vi "Calibration - Conductivity.vi"() -> ()   [LabVIEW 2016]
uses:
  calibration states.ctl
panel:
  in  "Highpoint":i32=1413 min=0
  in  "Lowpoint":i32=84 min=0
  in  "Calibrate3":bool
  out "Read indicator":bool
  out "Reading, uS/cm":dbl
  in  "Calibrate2":bool
  out "Status":string
  in  "Cancel":bool
  in  "Calibrate1":bool
  # "ATLAS SCIENTIFIC\nCONDUCTIVITY SENSOR CALIBRATION"
  # "Temperature has a significant effect on conductivity readings. The EZO Conductivity circuit has its temperature compensation set to 25C as the default. If the calibration solution is not within 5C of 25 C, check the temperature chart on the side of the calibration bottle, and calibrate to that value.\n\nLow point/single point calibration:\n1. Pour a small amount of the calibration solution into a cup. Shake the probe to make sure you do not have trapped air bubbles in the sensing area. \n2. You should see readings that are off by 1 – 40% from the stated value of the calibration solution. Wait for readings to stabilize (small movement from one reading to the next is normal).\n3. Once the readings stabilize, issue the \"Calibrate lowpoint\" command. Readings will NOT change - the calibration is not yet complete.\n\nHigh point calibration:\n1. Shake the probe to remove trapped air and adjust the temperature as done in the previous step.\n2. Once the readings have stabilized issue the \"Calibrate highpoint\" command. - Readings will change, calibration complete."
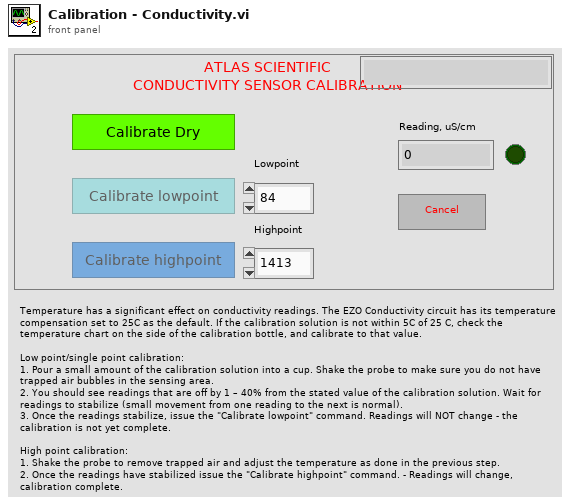
[diagram p1: front panel]
types:
  T1 = enum32{"Invalid", "Standard", "Closed", "Hidden", "Minimized", "Maximized"}
  T2 = typedef "Visa com cluster def (subVI).ctl" = cluster{"Sensor":string, "VISA resource name":refnum<visa-resource-name>, "error in/out":errorcluster, "bytes read":u32, "Com found ?":bool}
  T3 = typedef "calibration states.ctl" = string
  T4 = enum8{"Enabled", "Disabled", "Disabled and Grayed Out"}
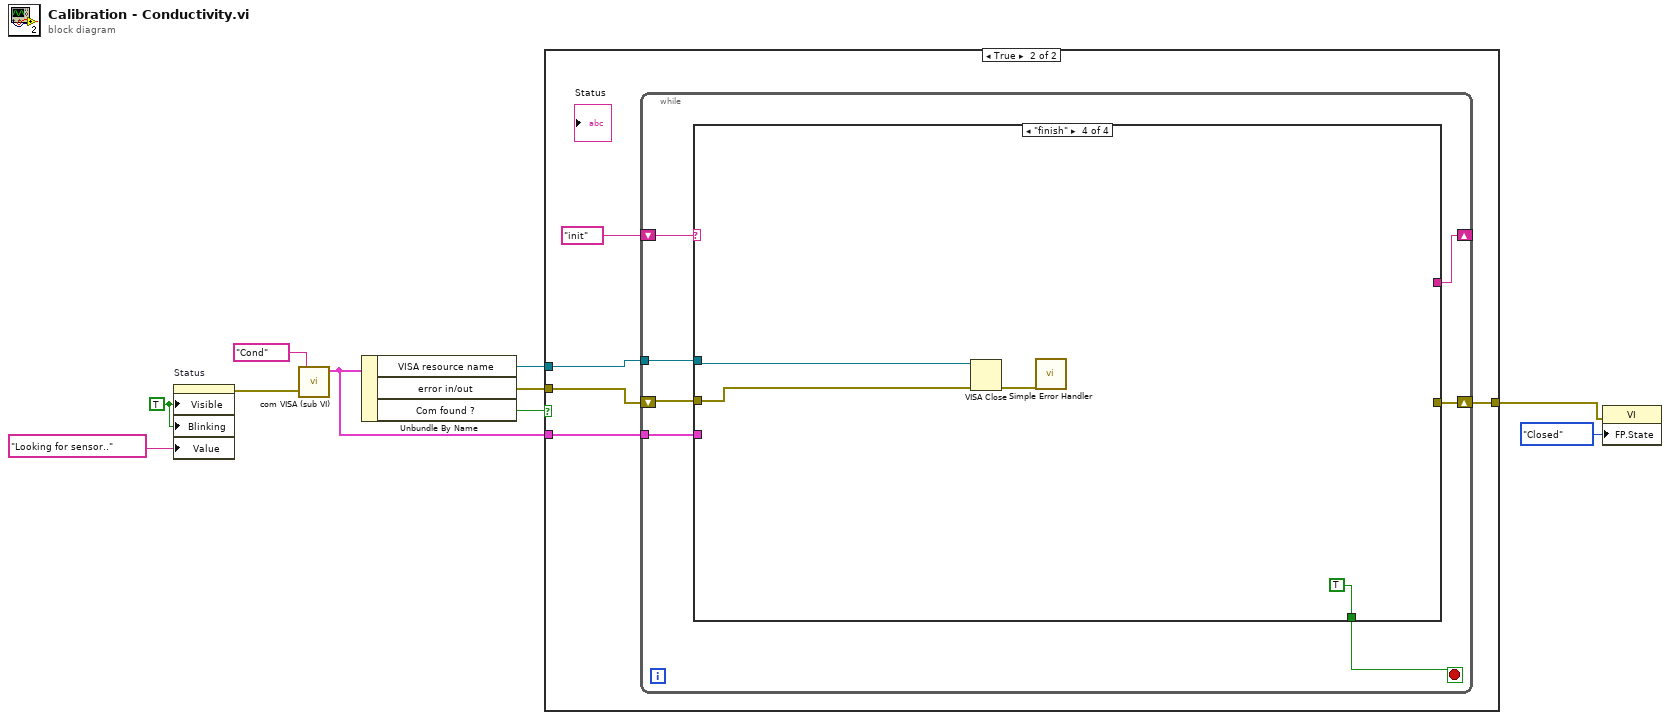
[diagram p0: block diagram]
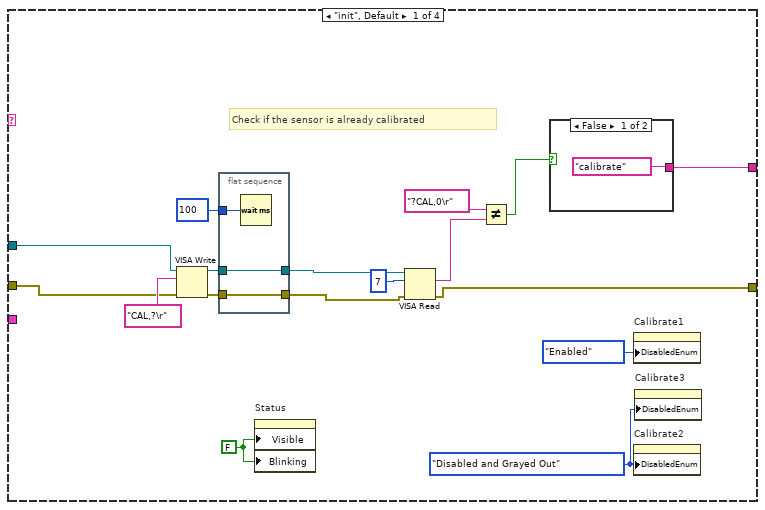
[diagram p3: hidden frame]
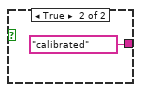
[diagram p4: hidden frame]
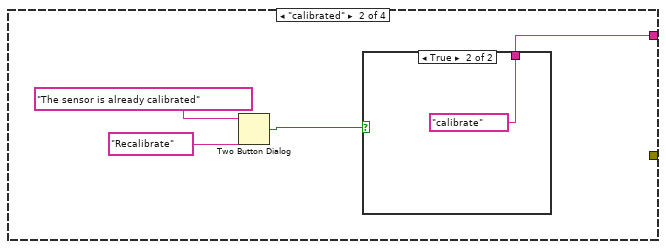
[diagram p5: hidden frame]
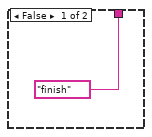
[diagram p6: hidden frame]
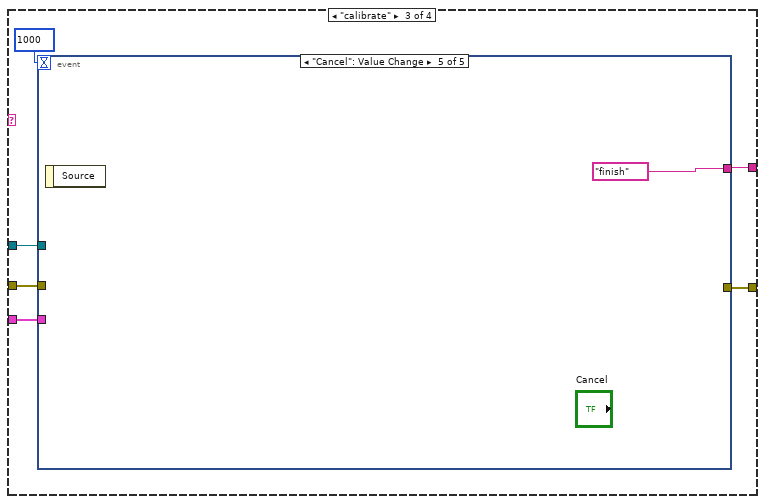
[diagram p7: hidden frame]
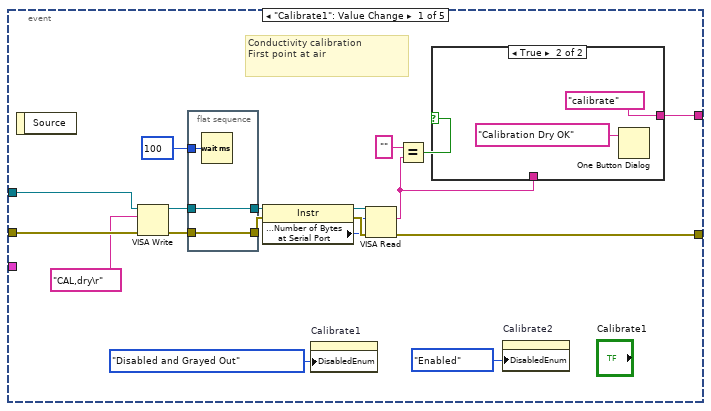
[diagram p8: hidden frame]
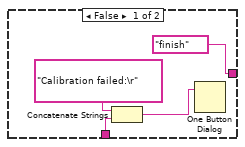
[diagram p9: hidden frame]
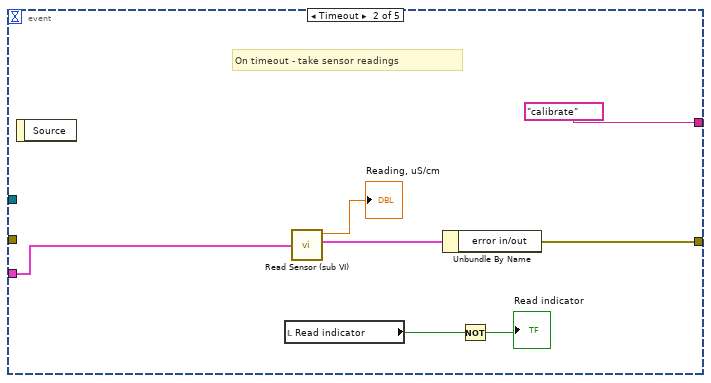
[diagram p10: hidden frame]
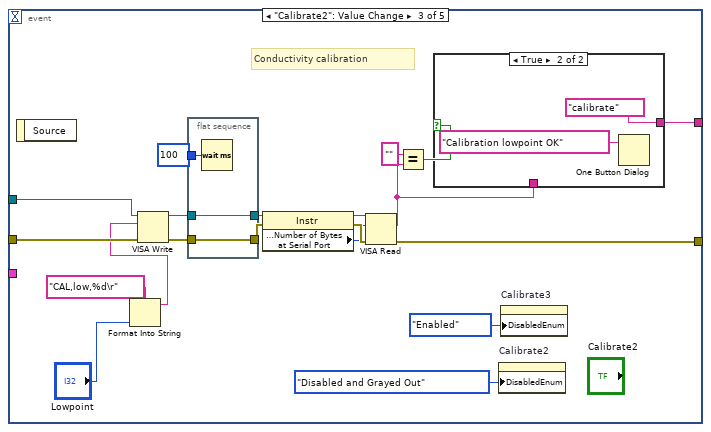
[diagram p11: hidden frame]
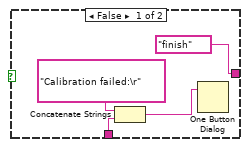
[diagram p12: hidden frame]
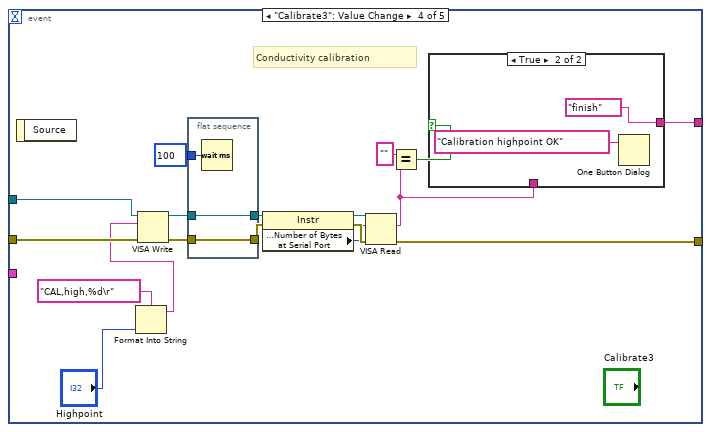
[diagram p13: hidden frame]
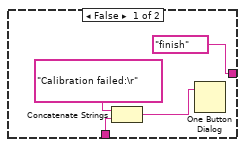
[diagram p14: hidden frame]
diagram:
  w10 = TRUE ("Visible")
  n1 = property on="Status" class="Str"("Visible"=w10, "Blinking"=w10, "Value"="Looking for sensor.." ("Status")) -> (error out=w6:errorcluster)  [unwired: 2 in, 1 out]
  n2 = call "com VISA (sub VI).vi"("Sensor"="Cond", "entrée d'erreur (pas d'erreur)"=w6) -> ("Output cluster"=w5:T2)  [unwired: 2 in, 1 out]
  n3 = Unbundle By Name(w5) -> ("VISA resource name"=w8:refnum<visa-resource-name>, "error in/out"=w7:errorcluster, "Com found ?"=w1:bool)
  n4 = case shown="True" w1 {
    tunnel: w8 -> [_ w14]
    tunnel: w7 -> [_ w13]
    tunnel: w5 -> [_ w12]
    tunnel: [_ w11] -> w2
    frame False {
    }
    frame True {
      n5 = while {
        tunnel: w14 -> [w21]
        shift-right: [w20] -> _
        shift-left: T3 "init" ("State Calibr") -> [w22]
        shift-right: [w18] -> w11
        shift-left: w13 -> [w19]
        tunnel: w12 -> [w17]
        stop <- w16 stop-if-true
        n6 = case shown="\"finish\"" w22 {
          tunnel: w21 -> [w31 _ w56 w149]
          tunnel: [w29 w45 w55 _] -> w20
          tunnel: [_ _ _ TRUE] -> w16
          tunnel: w19 -> [w27 _ w54 w148]
          tunnel: [w26 _ w53 _] -> w18
          tunnel: w17 -> [_ _ w51 _]
          frame "init", Default {
            w23 = T4."Disabled and Grayed Out" ("Disabled")
            w25 = FALSE ("Visible")
            # "Check if the sensor is already calibrated"
            n7 = VISA Write(VISA resource name=w31, write buffer="CAL,?\r", error in (no error)=w27) -> (VISA resource name out=w33:refnum<visa-resource-name>, error out=w32:errorcluster)  [unwired: 1 out]
            n8 = flat-sequence {
              tunnel: w32 -> [w43]
              tunnel: [w43] -> w37
              tunnel: w33 -> [w42]
              tunnel: [w42] -> w39
              tunnel: u32 100 ("delay before read (ms)") -> [w44]
              frame #0 {
                n9 = Wait (ms)(milliseconds to wait=w44) -> ()  [unwired: 1 out]
              }
            }
            n10 = property on="Status" class="Str"("Visible"=w25, "Blinking"=w25) -> ()  [unwired: 2 in, 2 out]
            n11 = VISA Read(VISA resource name=w39, byte count=u32 7, error in (no error)=w37) -> (read buffer=w28:string, error out=w26:errorcluster)  [unwired: 2 out]
            n12 = Not Equal?(x="?CAL,0\r" ("Response 2"), y=w28) -> (x != y?=w30:bool)
            n13 = case shown="False" w30 {
              tunnel: [T3 "calibrate" ("State Calibr") T3 "calibrated" ("State Calibr")] -> w29
              frame False {
              }
              frame True {
              }
            }
            n14 = property on="Calibrate1" class="Bool"("DisabledEnum"=T4."Enabled" ("Disabled")) -> ()  [unwired: 2 in, 2 out]
            n15 = property on="Calibrate2" class="Bool"("DisabledEnum"=w23) -> ()  [unwired: 2 in, 2 out]
            n16 = property on="Calibrate3" class="Bool"("DisabledEnum"=w23) -> ()  [unwired: 2 in, 2 out]
          }
          frame "calibrated" {
            n17 = Two Button Dialog(message="The sensor is already calibrated", 2:"Recalibrate" ("T button name (\"OK\")")) -> (T button?=w46:bool)  [unwired: 1 in]
            n18 = case shown="True" w46 {
              tunnel: [T3 "finish" ("State Calibr") T3 "calibrate" ("State Calibr")] -> w45
              frame False {
              }
              frame True {
              }
            }
          }
          frame "calibrate" {
            n19 = event shown="[4] \"Cancel\": Value Change" {
              selector: _ -> [_ _ _ _ _]
              dyn-events: _ -> [_ _ _ _ _]
              timeout: 1000 -> [_ _ _ _ _]
              tunnel: w56 -> [w70 _ w106 w133 _]
              tunnel: [w64 T3 "calibrate" ("State Calibr") w100 w127 T3 "finish" ("State Calibr")] -> w55
              tunnel: w54 -> [w61 _ w97 w124 _]
              tunnel: [w60 w84 w96 w123 _] -> w53
              tunnel: w51 -> [_ w86 _ _ _]
              event "Calibrate1": Value Change {
                # "Conductivity calibration\nFirst point at air"
                n20 = event-data() -> ()  [unwired: 1 in, 1 out]
                n21 = VISA Write(VISA resource name=w70, write buffer="CAL,dry\r" ("format string"), error in (no error)=w61) -> (VISA resource name out=w73:refnum<visa-resource-name>, error out=w74:errorcluster)  [unwired: 1 out]
                n22 = flat-sequence {
                  tunnel: w74 -> [w76]
                  tunnel: [w76] -> w66
                  tunnel: w73 -> [w75]
                  tunnel: [w75] -> w65
                  tunnel: u32 100 ("delay before read (ms)") -> [w77]
                  frame #0 {
                    n23 = Wait (ms)(milliseconds to wait=w77) -> ()  [unwired: 1 out]
                  }
                }
                n24 = property class="Instr"(reference=w65, error in=w66) -> (reference out=w69:refnum<visa-resource-name>, error out=w68:errorcluster, "Serial Settings:Number of Bytes at Serial Port"=w67:u32)
                n25 = property on="Calibrate1" class="Bool"("DisabledEnum"=T4."Disabled and Grayed Out" ("Disabled")) -> ()  [unwired: 2 in, 2 out]
                n26 = VISA Read(VISA resource name=w69, byte count=w67, error in (no error)=w68) -> (read buffer=w62:string, error out=w60:errorcluster)  [unwired: 2 out]
                n27 = Equal?(x="" ("Response 2"), y=w62) -> (x = y?=w63:bool)
                n28 = case shown="True" w63 {
                  tunnel: [T3 "finish" ("State Calibr") T3 "calibrate" ("State Calibr")] -> w64
                  tunnel: w62 -> [w80 _]
                  frame False {
                    n29 = Concatenate Strings("Calibration failed:\r" ("message"), w80) -> (w78:string)
                    n30 = One Button Dialog(message=w78) -> ()  [unwired: 1 in, 1 out]
                  }
                  frame True {
                    n31 = One Button Dialog(message="Calibration Dry OK") -> ()  [unwired: 1 in, 1 out]
                  }
                }
                n32 = property on="Calibrate2" class="Bool"("DisabledEnum"=T4."Enabled" ("Disabled")) -> ()  [unwired: 2 in, 2 out]
              }
              event Timeout {
                # "On timeout - take sensor readings"
                n33 = event-data() -> ()  [unwired: 1 in, 1 out]
                n34 = local read "Read indicator"() -> (w88:bool)
                n35 = call "Read Sensor (sub VI).vi"("Input cluster"=w86) -> ("Reading"=→"Reading, uS/cm":dbl, "Output cluster"=w85:T2)  [unwired: 2 in]
                n36 = Unbundle By Name(w85) -> ("error in/out"=w84:errorcluster)
                n37 = Not(x=w88) -> (.not. x?=→"Read indicator":bool)
              }
              event "Calibrate2": Value Change {
                # "Conductivity calibration"
                n38 = event-data() -> ()  [unwired: 1 in, 1 out]
                n39 = Format Into String(format string="CAL,low,%d\r", "Lowpoint") -> (resulting string=w93:string)  [unwired: 2 in, 1 out]
                n40 = VISA Write(VISA resource name=w106, write buffer=w93, error in (no error)=w97) -> (VISA resource name out=w109:refnum<visa-resource-name>, error out=w110:errorcluster)  [unwired: 1 out]
                n41 = flat-sequence {
                  tunnel: w110 -> [w112]
                  tunnel: [w112] -> w102
                  tunnel: w109 -> [w111]
                  tunnel: [w111] -> w101
                  tunnel: u32 100 ("delay before read (ms)") -> [w113]
                  frame #0 {
                    n42 = Wait (ms)(milliseconds to wait=w113) -> ()  [unwired: 1 out]
                  }
                }
                n43 = property class="Instr"(reference=w101, error in=w102) -> (reference out=w105:refnum<visa-resource-name>, error out=w104:errorcluster, "Serial Settings:Number of Bytes at Serial Port"=w103:u32)
                n44 = VISA Read(VISA resource name=w105, byte count=w103, error in (no error)=w104) -> (read buffer=w98:string, error out=w96:errorcluster)  [unwired: 2 out]
                n45 = Equal?(x="" ("Response 2"), y=w98) -> (x = y?=w99:bool)
                n46 = case shown="True" w99 {
                  tunnel: [T3 "finish" ("State Calibr") T3 "calibrate" ("State Calibr")] -> w100
                  tunnel: w98 -> [w116 _]
                  frame False {
                    n47 = Concatenate Strings("Calibration failed:\r" ("message"), w116) -> (w114:string)
                    n48 = One Button Dialog(message=w114) -> ()  [unwired: 1 in, 1 out]
                  }
                  frame True {
                    n49 = One Button Dialog(message="Calibration lowpoint OK") -> ()  [unwired: 1 in, 1 out]
                  }
                }
                n50 = property on="Calibrate2" class="Bool"("DisabledEnum"=T4."Disabled and Grayed Out" ("Disabled")) -> ()  [unwired: 2 in, 2 out]
                n51 = property on="Calibrate3" class="Bool"("DisabledEnum"=T4."Enabled" ("Disabled")) -> ()  [unwired: 2 in, 2 out]
              }
              event "Calibrate3": Value Change {
                # "Conductivity calibration"
                n52 = event-data() -> ()  [unwired: 1 in, 1 out]
                n53 = Format Into String(format string="CAL,high,%d\r", "Highpoint") -> (resulting string=w120:string)  [unwired: 2 in, 1 out]
                n54 = VISA Write(VISA resource name=w133, write buffer=w120, error in (no error)=w124) -> (VISA resource name out=w136:refnum<visa-resource-name>, error out=w137:errorcluster)  [unwired: 1 out]
                n55 = flat-sequence {
                  tunnel: w137 -> [w139]
                  tunnel: [w139] -> w129
                  tunnel: w136 -> [w138]
                  tunnel: [w138] -> w128
                  tunnel: u32 100 ("delay before read (ms)") -> [w140]
                  frame #0 {
                    n56 = Wait (ms)(milliseconds to wait=w140) -> ()  [unwired: 1 out]
                  }
                }
                n57 = property class="Instr"(reference=w128, error in=w129) -> (reference out=w132:refnum<visa-resource-name>, error out=w131:errorcluster, "Serial Settings:Number of Bytes at Serial Port"=w130:u32)
                n58 = VISA Read(VISA resource name=w132, byte count=w130, error in (no error)=w131) -> (read buffer=w125:string, error out=w123:errorcluster)  [unwired: 2 out]
                n59 = Equal?(x="" ("Response 2"), y=w125) -> (x = y?=w126:bool)
                n60 = case shown="True" w126 {
                  tunnel: [T3 "finish" ("State Calibr") T3 "finish" ("State Calibr")] -> w127
                  tunnel: w125 -> [w143 _]
                  frame False {
                    n61 = Concatenate Strings("Calibration failed:\r" ("message"), w143) -> (w141:string)
                    n62 = One Button Dialog(message=w141) -> ()  [unwired: 1 in, 1 out]
                  }
                  frame True {
                    n63 = One Button Dialog(message="Calibration highpoint OK") -> ()  [unwired: 1 in, 1 out]
                  }
                }
              }
              event "Cancel": Value Change {
                n64 = event-data() -> ()  [unwired: 1 in, 1 out]
              }
            }
          }
          frame "finish" {
            n65 = VISA Close(VISA resource name=w149, error in (no error)=w148) -> (error out=w150:errorcluster)
            n66 = call <vilib>:"Simple Error Handler.vi"("error in (no error)"=w150) -> ()  [unwired: 1 in, 8 out]
          }
        }
      }
    }
  }
  n67 = property class="VI"(error in=w2, "FP.State"=T1."Closed" ("Front Panel Window:State")) -> ()  [unwired: 1 in, 2 out]
